vi "Toggle Remote Mode.vi"(8 "error in (no error)":errorcluster, 10 "Remote":bool, 11 "IF_XX in":refnum<class "IF_XX.lvclass">) -> (0 "error out":errorcluster, 3 "IF_XX out":refnum<class "IF_XX.lvclass">)   [LabVIEW 2019, in "IF_XX.lvlib" / "IF_XX.lvclass"]
doc: "This toggles the power supply between remote and local operation.\n\nThe channel select function is unclear, so I have left it defaulted to Auto for now. The notes show that the channel needs to be selected only on the first call, so we'll have to see what we see."
uses:
  Library/IF_XX.lvclass
  Library/IF_XX.lvclass/IF_XX.ctl
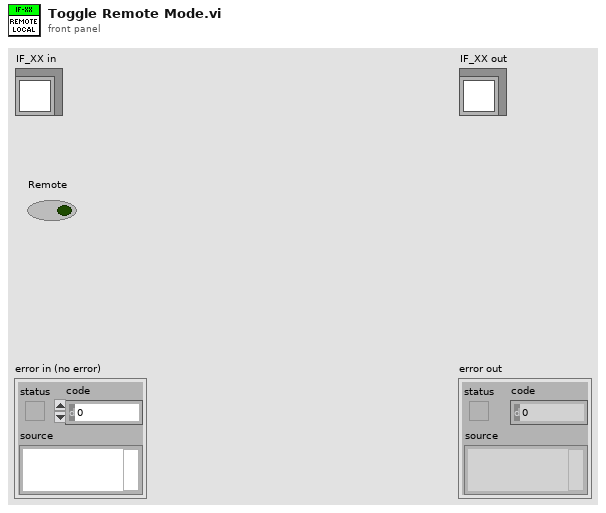
[diagram p1: front panel]
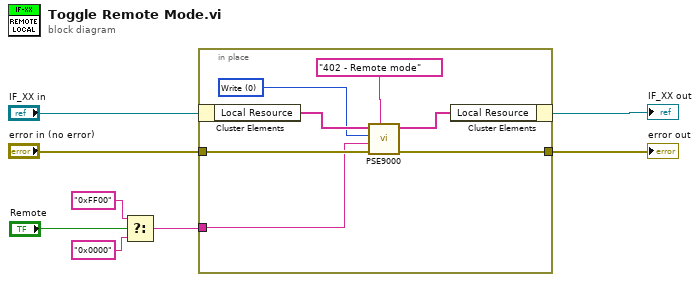
[diagram p0: block diagram]
diagram:
  n1 = Select(t="0xFF00" ("Value"), s="Remote", f="0x0000" ("Value")) -> (s? t:f=w1:string)
  n2 = in-place {
    in-place-border: "error in (no error)" -> [w13]
    in-place-border: [w12] -> w6
    in-place-border: w1 -> [w9]
    w10 = u8 0 items=["Write", "Read"] ("Access")
    n3 = in-place-cluster #1("IF_XX in") -> ("Local Resource"=w15:string[])
    n4 = call <instrlib>:"PSE9000.vi"("Command list"="402 - Remote mode", "Error in"=w13, "Value"=w9, "Access"=w10, "Device information in"=w15) -> ("Error out"=w12:errorcluster, "Device information out"=w14:string[])  [unwired: 1 in, 2 out]
    n5 = in-place-cluster #1("Local Resource"=w14) -> (→"IF_XX out":refnum<class "IF_XX.lvclass">)
  }
  "error out" <- w6
